vi "Handle Error.vi"(8 "error in (no error)":errorcluster, 11 "4503 in":refnum<class "4503.lvclass">) -> (0 "error out":errorcluster, 2 "stop actor?":bool=TRUE, 3 "4503 out":refnum<class "4503.lvclass">)   [LabVIEW 2024, in "4503 Actor.lvlib" / "4503.lvclass"]
doc: "(<B>Filename</B>: Actor Framework.lvlib:Actor.lvclass:Handle Error.vi)\n\nDefines how the actor handles an error that occurred while processing a message. By default, this method does nothing except stop the actor."
uses:
  4503.lvclass
  <vilib>/ActorFramework/Actor/Actor.lvclass
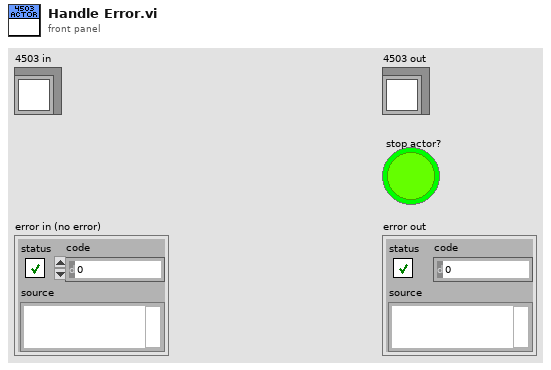
[diagram p1: front panel]
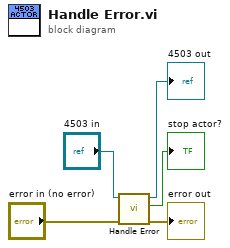
[diagram p0: block diagram]
diagram:
  n1 = call-parent "Handle Error.vi"("error in (no error)"="error in (no error)", "Actor in"="4503 in") -> ("error out"=→"error out":errorcluster, "stop actor?"=→"stop actor?":bool, "Actor out"=→"4503 out":refnum<class "4503.lvclass">)  [unwired: 7 in]
